vi "get_env_variable.vi"(3 "Environment Variable Name":string) -> (0 "error out":errorcluster, 1 "Value":string)   [LabVIEW 2020, in "env_variables.lvlib"]
uses:
  env_variables.lvlib
  <vilib>/Utility/config.llb/Read Key (String).vi
  <vilib>/Utility/config.llb/NI_LVConfig.lvlib
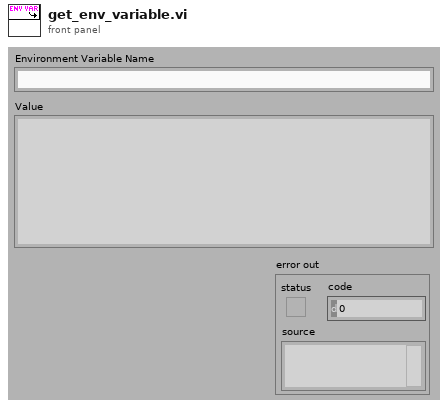
[diagram p1: front panel]
types:
  T1 = typedef "NI_LVConfig.lvlib/Config Data RefNum.ctl" = refnum<k1>
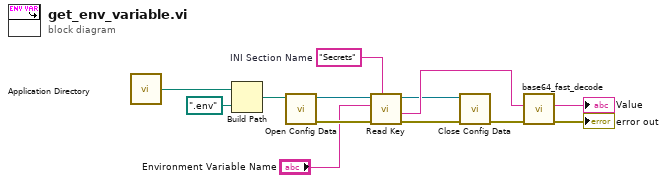
[diagram p0: block diagram]
diagram:
  w10 = "Secrets"  # INI Section Name
  n1 = call <vilib>:"Application Directory.vi"() -> ("Application Directory"=w13:path)
  n2 = Build Path(base path=w13, name or relative path=path ".env") -> (appended path=w11:path)
  n3 = call <vilib>:"Open Config Data.vi"("configuration file path"=w11) -> ("error out"=w9:errorcluster, "refnum"=w8:T1)  [unwired: 8 in, 1 out]
  n4 = call-poly <vilib>:"Read Key.vi"("section"=w10, "error in (no error)"=w9, "key"="Environment Variable Name", "refnum"=w8) -> ("error out"=w4:errorcluster, "value"=w6:string, "refnum out"=w3:T1)  [unwired: 4 in, 1 out]
  n5 = call <vilib>:"Close Config Data.vi"("error in (no error)"=w4, "refnum"=w3) -> ("error out"=w2:errorcluster)  [unwired: 8 in, 1 out]
  n6 = call "base64_fast_decode.vi"("error in (no error)"=w2, "string in (base64-encoded)"=w6) -> ("error out"=→"error out":errorcluster, "string out (decoded)"=→"Value":string)  [unwired: 8 in]
